vi "CRYCalc RunIndex.vi"(1 "No.VI":i32) -> (9 "Out Index":i16)   [LabVIEW 2013]
uses:
  CRYStatistics Global.vi
  Task Sequence/CRYProject Run Control Global.vi
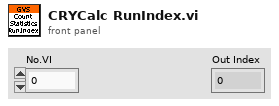
[diagram p1: front panel]
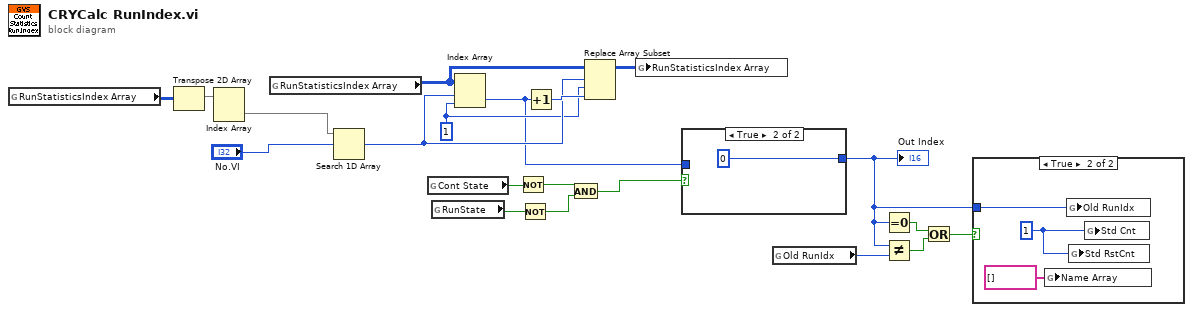
[diagram p0: block diagram]
diagram:
  w17 = 1 ("disabled index (col)")
  n1 = global read "CRYStatistics Global.vi" "RunStatisticsIndex Array"() -> (w20:u16[][])
  n2 = Transpose 2D Array(2D array=w20) -> (transposed array=w14:u16[][])
  n3 = Index Array(array=w14) -> (element=w13:u16[])  [unwired: 2 in]
  n4 = global read "CRYStatistics Global.vi" "RunStatisticsIndex Array"() -> (w16:u16[][])
  n5 = Search 1D Array(1D array=w13, element="No.VI") -> (index of element=w18:i32)  [unwired: 1 in]
  n6 = global read "CRYProject Run Control Global.vi" "Cont State"() -> (w11:bool)
  n7 = global read "CRYProject Run Control Global.vi" "RunState"() -> (w10:bool)
  n8 = Index Array(array=w16, index (row)=w18, index (col)=w17) -> (element=w6:u16)
  n9 = Not(x=w11) -> (.not. x?=w9:bool)
  n10 = Not(x=w10) -> (.not. x?=w8:bool)
  n11 = Increment(x=w6) -> (x+1=w19:u16)
  n12 = And(x=w9, y=w8) -> (x .and. y?=w7:bool)
  n13 = Replace Array Subset(array=w16, new element=w19, index (row)=w18, index (col)=w17) -> (w15:u16[][])
  n14 = global write "CRYStatistics Global.vi" "RunStatisticsIndex Array"(w15) -> ()
  n15 = case shown="True" w7 {
    tunnel: [w21 u16 0 ("Calculated Rst 2")] -> w1
    tunnel: w6 -> [w21 _]
    frame False {
    }
    frame True {
    }
  }
  "Out Index" <- w1
  n16 = global read "CRYStatistics Global.vi" "Old RunIdx"() -> (w5:u32)
  n17 = Equal To 0?(x=w1) -> (x = 0?=w4:bool)
  n18 = Not Equal?(x=w1, y=w5) -> (x != y?=w3:bool)
  n19 = Or(x=w4, y=w3) -> (x .or. y?=w2:bool)
  n20 = case shown="True" w2 {
    tunnel: w1 -> [_ w24]
    frame False {
    }
    frame True {
      w23 = u32 1 ("Std Cnt")
      n21 = global write "CRYStatistics Global.vi" "Name Array"(string[] [] ("Name Array")) -> ()
      n22 = global write "CRYStatistics Global.vi" "Old RunIdx"(w24) -> ()
      n23 = global write "CRYStatistics Global.vi" "Std RstCnt"(w23) -> ()
      n24 = global write "CRYStatistics Global.vi" "Std Cnt"(w23) -> ()
    }
  }
